vi "GetGlobalVariables.vi"() -> ()   [LabVIEW 2019]
panel:
  out "data":string
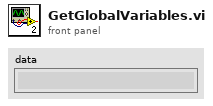
[diagram p1: front panel]
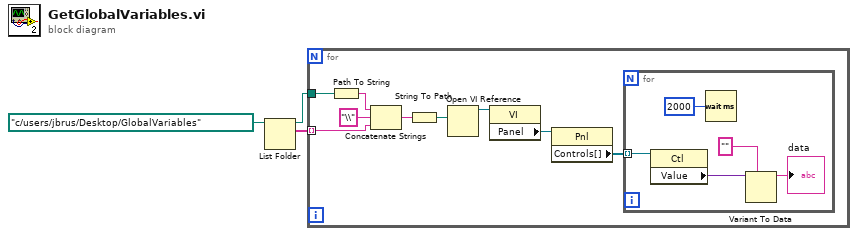
[diagram p0: block diagram]
diagram:
  n1 = List Folder(path=path "c:/users/jbrus/Desktop/GlobalVariables" ("vi path")) -> (path out=w1:path, filenames=w2:string[])  [unwired: 3 in, 2 out]
  n2 = for {
    tunnel: w2 -> [w7] mode=indexing
    tunnel: w1 -> [w9]
    n3 = Path To String(path=w9) -> (string=w8:string)
    n4 = Concatenate Strings(w8, "\\" ("string"), w7) -> (w5:string)
    n5 = String To Path(string=w5) -> (path=w4:path)
    n6 = Open VI Reference(vi path=w4) -> (vi reference=w11:refnum<vi>)  [unwired: 5 in, 1 out]
    n7 = property class="VI"(reference=w11) -> ("Panel"=w10:refnum<vi>)  [unwired: 1 in, 2 out]
    n8 = property class="Pnl"(reference=w10) -> ("Controls[]"=w12:refnum<vi>[])  [unwired: 1 in, 2 out]
    n9 = for {
      tunnel: w12 -> [w16] mode=indexing
      n10 = property class="Ctl"(reference=w16) -> ("Value"=w15:variant)  [unwired: 1 in, 2 out]
      n11 = Wait (ms)(milliseconds to wait=u32 2000) -> ()  [unwired: 1 out]
      n12 = Variant To Data(type="", Variant=w15) -> (data=→"data":string)  [unwired: 1 in, 1 out]
    }
  }
